vi "Scan_Hopping_CV_VUW.vi"() -> ()   [LabVIEW 2023]
uses:
  Sub_Vi/TypeDefs/Settings.ctl
  Sub_Vi/TypeDefs/ChangeOnFly.ctl
  Sub_Vi/TypeDefs/Display.ctl
  Settings.vi
panel:
  in  "Feedback Threshold \nGreater Than (Amps)":dbl=-1e-09
  in  "StopCond_GreaterThan? 2":bool
  in  "NumberOfCVsAtEachPoint":i32=1
  in  "Hopping Distance Between Lines (um)":dbl=1.0
  in  "Pre CV HoldTime /s":dbl format="%#_13g"
  in  "CV Rate / V/s":dbl=0.2
  in  "Voltage to Electrode (V) 3":dbl=-2.0
  in  "Voltage to Electrode (V) 2":dbl=1.0
  in  "Display Cluster":T1
  in  "ChangeonFly":T2
  in  "SettingsCluster":T3={"Sample Rate (us)"=1, "Samples Per Data Point (int, power of 2)"=1000, "DistanceToBulk (um)"=-1.0, "HoldTimeScaler"=40000, "SaveData"=TRUE, "DistanceToBulk (um) 2"=-1.0, "DistanceToBulk (um) 3"=-1.0}
  in  "Feedback Type":T4(ring)=enum."Current 1"
  in  "StopCond_GreaterThan?":bool=TRUE
  in  "Approach Rate Hopping (um/s)":dbl=0.15
  in  "Retract Rate (um/s)":dbl=1.0
  in  "Hopping Distance Along Line(um)":dbl=1.0
  in  "Z End (um)":dbl
  in  "Distance To Retract (um)":dbl=5.0
  in  "Upper dZ limit":i32=8
  in  "Feedback Threshold \nLess Than (Amps)":dbl=1e-09
  in  "P":fxp<+/-,32,1>=0.029999999795109034 format="%.32g"
  in  "X Center (um)":dbl=100.0 min=0.0 max=300.0
  in  "Y Center (um)":dbl=100.0 min=0.0 max=300.0
  in  "Y Width (um)":dbl=10.0
  in  "X Width (um)":dbl=10.0
  in  "Lateral Movement Rate (um/s)":dbl=5.0
  in  "Voltage to Electrode (V)":dbl=-0.4
  in  "Approach Rate (um/s)":dbl=0.5
  in  "Z Start height (um)":dbl=150.0
  in  "Start scan Button":bool
  in  "Stop":bool
  in  "Pause":bool
  out "Y end":dbl
  out "X end":dbl
  out "X start":dbl
  out "Y start":dbl
  in  "Tab Control 4":T5(tab)=enum."AC Approach 2"
  out "Topology":dbl[][](graph)
  out "Current 1":dbl[][](graph)
  out "Current 2":dbl[][](graph)
  out "Current 3":dbl[][](graph)
  out "V vs C1":cluster{"Y":dbl[], "Y":dbl[]}[](graph)
  out "Z vs C3":cluster{"Y":dbl[], "Y":dbl[]}[](graph)
  out "Lock in Phase":dbl[](graph)
  out "Lock in amp":dbl[](graph)
  out "t vs C2":dbl[](graph)
  out "t vs C1":dbl[](graph)
  out "Z vs C1":cluster{"Y":dbl[], "Y":dbl[]}[](graph)
  # "Approach  Settings"
  # "Feedback  Settings"
  # "Hopping Settings"
  # "CV"
  # "Scan  Area"
  # "Define Scan area \nAbout centre"
  # "Change top/bottom values \ndepending on scan"
  # "Change top/bottom values \ndepending on scan"
  # "Change top/bottom values \ndepending on scan"
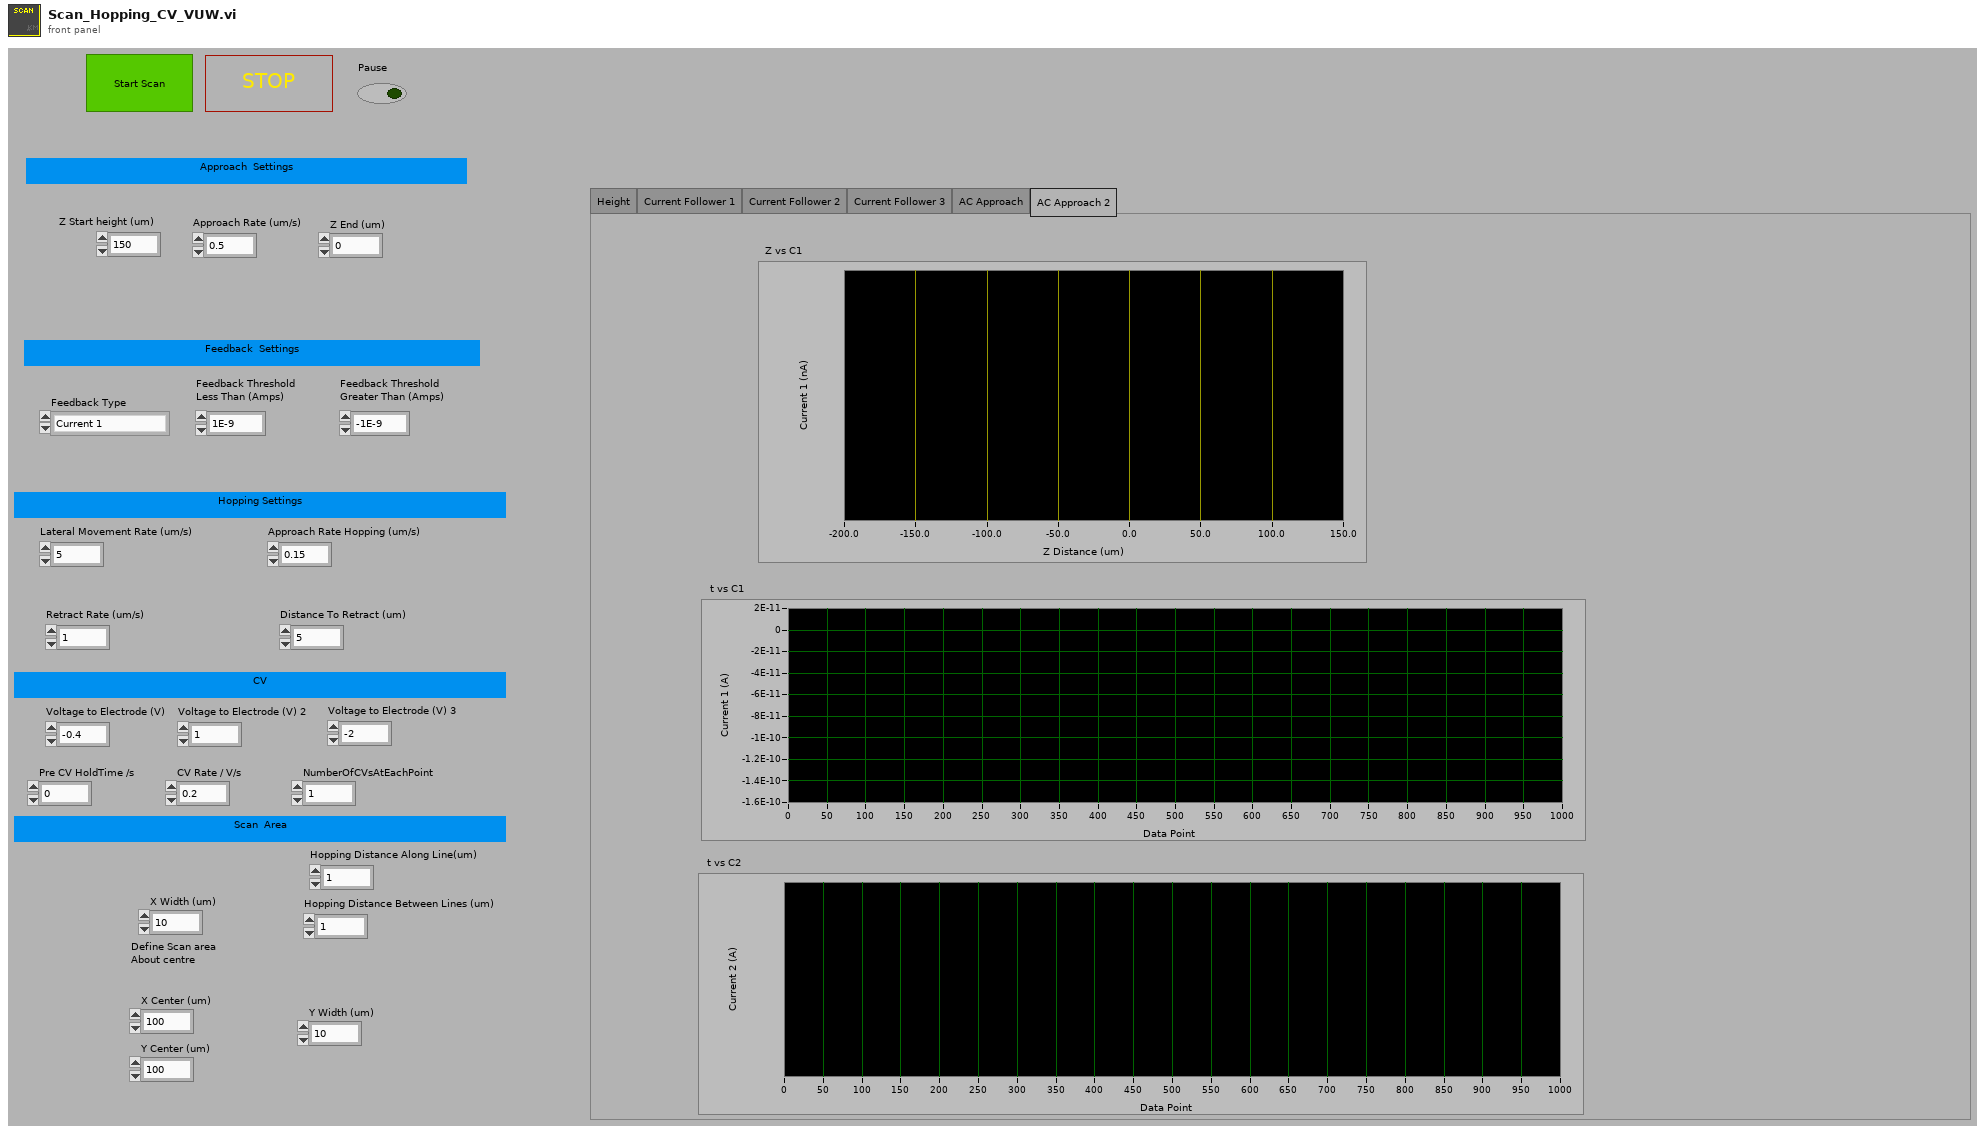
[diagram p1: front panel]
types:
  T1 = typedef "Display.ctl" = cluster{"X":refnum<vi>, "Y":refnum<vi>, "Z":refnum<vi>, "Amp":refnum<vi>, "Phase":refnum<vi>, "t vs Z":refnum<vi>, "t vs C1":refnum<vi>, "t vs C2":refnum<vi>, "t vs C3":refnum<vi>, "t vs Amp":refnum<vi>, "t vs Phase":refnum<vi>, "t vs X":refnum<vi>, "t vs Y":refnum<vi>, "Z vs C1":refnum<vi>, "Z vs C2":refnum<vi>, "Z vs C3":refnum<vi>, "V vs C1":refnum<vi>, "V vs C2":refnum<vi>, "V vs C3":refnum<vi>, "X/Y/Z F":refnum<vi>, "X/Y/Z R":refnum<vi>, "X/Y/C1 F":refnum<vi>, "X/Y/C1 R":refnum<vi>, "X/Y/C2 F":refnum<vi>, "X/Y/C2 R":refnum<vi>, "X/Y/C3 F":refnum<vi>, "X/Y/C3 R":refnum<vi>, "NumberOfLines":u16, "um Per Pixel":dbl, "um Per Line":dbl, "X Center":dbl, "Hop X/Y/Z":refnum<vi>, "Hop X/Y/C1":refnum<vi>, "Hop X/Y/C2":refnum<vi>, "Hop X/Y/C3":refnum<vi>, "X Width":dbl, "Y Width":dbl, "Hopping Distance":dbl, "V2 vs C1":refnum<vi>, "V vs Phase":refnum<vi>, "Y Center":dbl, "Number of Pixels":dbl, "V2 vs C2":refnum<vi>, "V2 vs C3":refnum<vi>, "V vs y":refnum<vi>, "V2 vs y":refnum<vi>, "Z vs Amp":refnum<vi>, "Z vs Phase":refnum<vi>}
  T2 = typedef "ChangeOnFly.ctl" = cluster{"Stop (boolean)":refnum<vi>, "Pause (boolean)":refnum<vi>, "EndCurrentLine (boolean)":refnum<vi>, "max movement per update step (Interger, nm)":refnum<vi>, "P (float, arb)":refnum<vi>, "Feedback set point (double, Amps)":refnum<vi>, "Voltage (double, V)":refnum<vi>, "Feedback set point 2 (double, Amps)":refnum<vi>, "Stop on Greater Than 2? (boolean)":refnum<vi>, "Stop on Greater Than? (boolean)":refnum<vi>, "Voltage 2 (double, V)":refnum<vi>, "Feedback Type (enum)":refnum<vi>, "Feedback Type 2 (enum)":refnum<vi>}
  T3 = typedef "Settings.ctl" = cluster{"Sample Rate (us)":u32, "Samples Per Data Point (int, power of 2)":i16, "DistanceToBulk (um)":dbl, "HoldTimeScaler":u64, "SaveData":bool, "DistanceToBulk (um) 2":dbl, "DistanceToBulk (um) 3":dbl}
  T4 = enum16{"AC Magnitude", "Current 1", "Current 2", "Phase"}
  T5 = enum32{"Height", "Current Follower 1", "Current Follower 2", "Current Follower 3", "AC Approach", "AC Approach 2"}
  T6 = cluster{"Scan Rate (um/s)":dbl, "X Start":dbl, "X End":dbl, "Y Start":dbl, "Y End":dbl, " Z Start":dbl, "HoppingDistance":dbl, "V":dbl, "Z End":dbl, "Approach Rate Hopping (um/s)":dbl, "Retrack Rate (um/s)":dbl, "V 2":dbl, "Approach Rate (um/s)":dbl, "V 3":dbl, "CV Rate / V/s":dbl, "V 4":dbl, "V 1":dbl, "HoldTime1/s":dbl, "Hold time 2 / s":dbl, "Hold time 3/ s":dbl, "HoppingDistanceBetweenLines":dbl}
  T7 = typedef "WayPointCluster.ctl" = cluster{"X (um)":dbl[], "Y (um)":dbl[], "Z (um)":dbl[], "V (V)":dbl[], "X Velocity (um s-1)":dbl[], "Y Velocity (um s-1)":dbl[], "Z Velocity (um s-1)":dbl[], "V Velocity (V s-1)":dbl[], "FeedBack Type (enum)":u16[], "Move X (boolean)":bool[], "Move Y (boolean)":bool[], "Move Z (boolean)":bool[], "Move V (boolean)":bool[], "Jump V (boolean)":bool[], "Hold (boolean)":bool[], "Hold Time":u32[], "V2 (V)":dbl[], "Move V2":bool[], "V2 Velocity (V s-1)":dbl[], "Jump V2 (boolean)":bool[], "Update z Position delta (ms)":i16[], "Hold Feedback1":bool[], "Move Z PicoMotor":bool[], " Z PicoMotor Direction":bool[], "DIO0":bool[]}
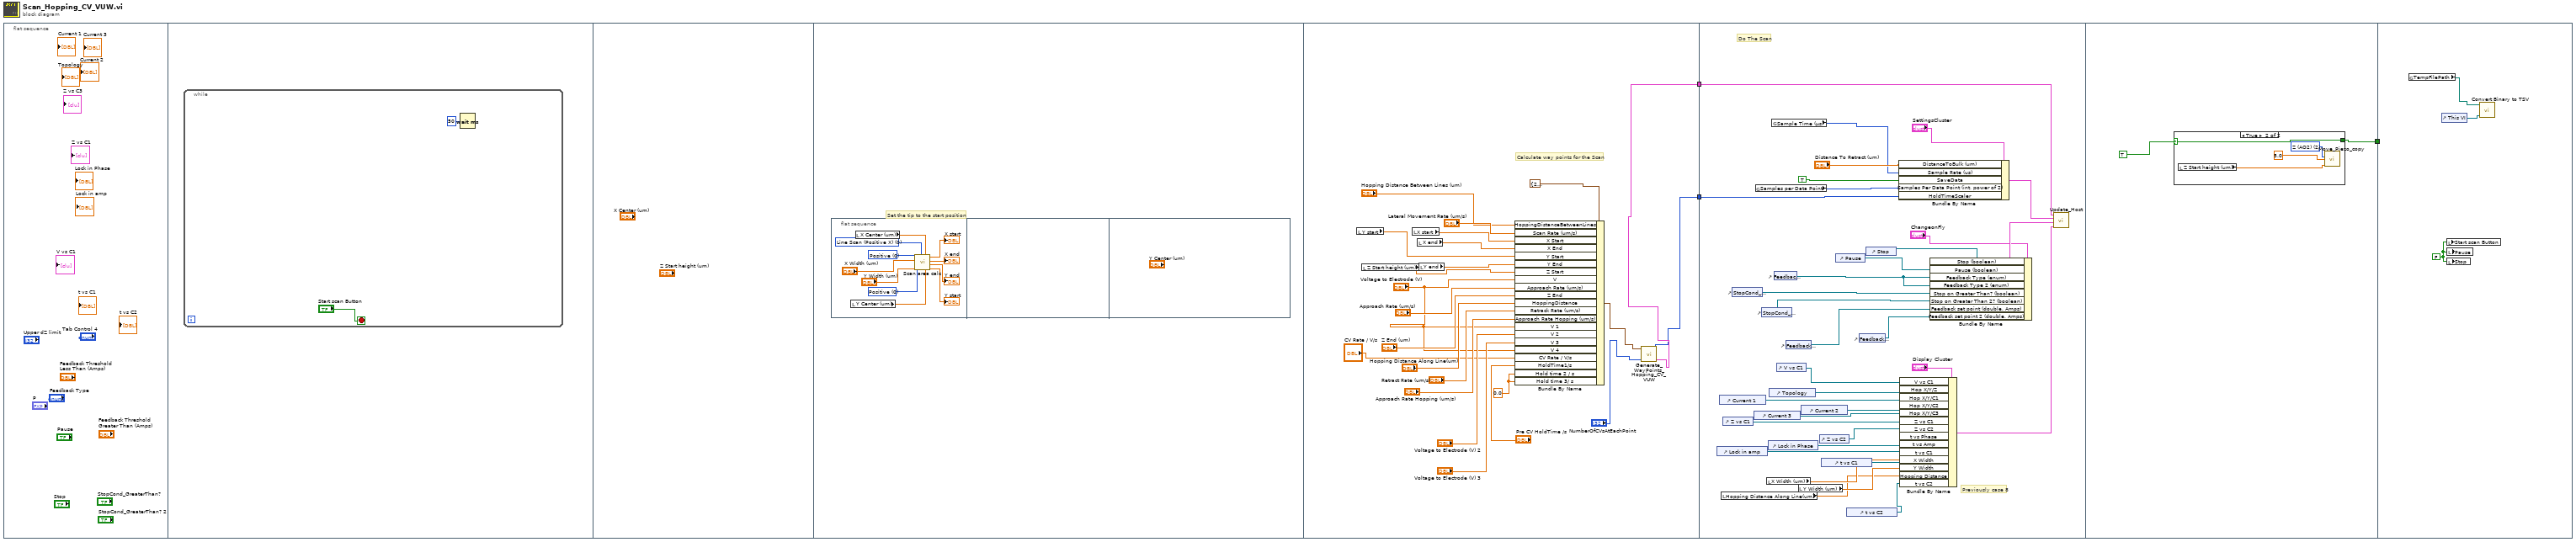
[diagram p0: block diagram]
diagram:
  n1 = flat-sequence {
    tunnel: [w18] -> w3
    tunnel: [w17] -> w1
    tunnel: w3 -> [w72]
    tunnel: w1 -> [w46]
    tunnel: [w73] -> w2
    tunnel: w2 -> [_]
    frame #0 {
    }
    frame #1 {
      n2 = while {
        stop <- "Start scan Button" stop-if-true
        n3 = Wait (ms)(milliseconds to wait=u32 50) -> ()  [unwired: 1 out]
      }
    }
    frame #2 {
    }
    frame #3 {
      # "Set the tip to the start position"
      n4 = flat-sequence {
        frame #0 {
          w6 = u16 0 items=["Positive", "Negative"] ("Major Axis Direction")
          w7 = u16 0 items=["Positive", "Negative"] ("Minor Axis Direction")
          w8 = u16 0 items=["Line Scan (Positive X)", "Line Scan (Negative X)", "Line Scan (Positive Y)", "Line Scan (Negative Y)"] ("Scan Type")
          n5 = local read "Y Center (um)"() -> (w9:dbl)
          n6 = local read "X Center (um)"() -> (w10:dbl)
          n7 = call "Scan area calc.vi"("Y Width"="Y Width (um)", "Major Axis Direction"=w6, "X Width"="X Width (um)", "Minor Axis Direction"=w7, "Scan Type"=w8, "Y Center"=w9, "X Center"=w10) -> ("Y start"=→"Y start":dbl, "Y end"=→"Y end":dbl, "X end"=→"X end":dbl, "X start"=→"X start":dbl)
        }
        frame #1 {
        }
        frame #2 {
        }
      }
    }
    frame #4 {
      w24 = 0.0 ("HoldTime1/s")
      # "Calculate way points for the Scan"
      n8 = local read "Y start"() -> (w29:dbl)
      n9 = local read "Z Start height (um)"() -> (w34:dbl)
      n10 = local read "X start"() -> (w39:dbl)
      n11 = local read "X end"() -> (w38:dbl)
      n12 = local read "Y end"() -> (w37:dbl)
      n13 = Bundle By Name(cluster=T6 {"Scan Rate (um/s)"=20.0, "X Start"=180.0, "X End"=220.0, "Y Start"=199.0, "Y End"=201.0, " Z Start"=0.0, "HoppingDistance"=0.5, "V"=0.0, "Z End"=38.0, "Approach Rate Hopping (um/s)"=0.5, "Retrack Rate (um/s)"=20.0, "V 2"=0.0, "Approach Rate (um/s)"=0.5, "V 3"=0.0, "CV Rate / V/s"=1.0, "V 4"=0.0, "V 1"=0.0, "HoldTime1/s"=0.5, "Hold time 2 / s"=0.0, "Hold time 3/ s"=0.0, "HoppingDistanceBetweenLines"=0.5} ("Input Cluster"), "HoppingDistanceBetweenLines"="Hopping Distance Between Lines (um)", "Scan Rate (um/s)"="Lateral Movement Rate (um/s)", "X Start"=w39, "X End"=w38, "Y Start"=w29, "Y End"=w37, "Z Start"=w34, "V"="Voltage to Electrode (V)", "Approach Rate (um/s)"="Approach Rate (um/s)", "Z End"="Z End (um)", "HoppingDistance"="Hopping Distance Along Line(um)", "Retrack Rate (um/s)"="Retract Rate (um/s)", "Approach Rate Hopping (um/s)"="Approach Rate Hopping (um/s)", "V 1"="Voltage to Electrode (V)", "V 2"="Voltage to Electrode (V) 2", "V 3"="Voltage to Electrode (V) 3", "V 4"="Voltage to Electrode (V)", "CV Rate / V/s"="CV Rate / V/s", "HoldTime1/s"="Pre CV HoldTime /s", "Hold time 2 / s"=w24, "Hold time 3/ s"=w24) -> (w19:T6)
      n14 = call "Generate_WayPoints_Hopping_CV_VUW.vi"("NumberOfCVsAtEachPoint"="NumberOfCVsAtEachPoint", "Input Cluster"=w19) -> ("output cluster"=w18:T7, "WaitTimeScaler"=w17:u64)  [unwired: 8 in]
    }
    frame #5 {
      # "Previously case 8"
      # "Do The Scan"
      n15 = control-ref of="Lock in amp"() -> (w65:refnum<vi>)
      n16 = control-ref of="Current 1"() -> (w59:refnum<vi>)
      n17 = local read "Hopping Distance Along Line(um)"() -> (w55:dbl)
      n18 = control-ref of="Z vs C1"() -> (w62:refnum<vi>)
      n19 = control-ref of="StopCond_GreaterThan?"() -> (w44:refnum<vi>)
      n20 = control-ref of="Current 3"() -> (w61:refnum<vi>)
      n21 = global read "Settings.vi" "Samples per Data Point"() -> (w51:u16)
      n22 = control-ref of="StopCond_GreaterThan? 2"() -> (w43:refnum<vi>)
      n23 = local read "X Width (um)"() -> (w57:dbl)
      n24 = control-ref of="Lock in Phase"() -> (w64:refnum<vi>)
      n25 = control-ref of="Topology"() -> (w58:refnum<vi>)
      n26 = global read "Settings.vi" "Sample Time (µs)"() -> (w48:u32)
      n27 = control-ref of="Feedback Type"() -> (w45:refnum<vi>)
      n28 = control-ref of="V vs C1"() -> (w49:refnum<vi>)
      n29 = control-ref of="Feedback Threshold \nLess Than (Amps)"() -> (w42:refnum<vi>)
      n30 = local read "Y Width (um)"() -> (w56:dbl)
      n31 = control-ref of="Current 2"() -> (w60:refnum<vi>)
      n32 = control-ref of="Z vs C2"() -> (w63:refnum<vi>)
      n33 = control-ref of="t vs C1"() -> (w66:refnum<vi>)
      n34 = control-ref of="Pause"() -> (w68:refnum<vi>)
      n35 = control-ref of="t vs C2"() -> (w40:refnum<vi>)
      n36 = control-ref of="Feedback Threshold \nGreater Than (Amps)"() -> (w41:refnum<vi>)
      n37 = control-ref of="Stop"() -> (w67:refnum<vi>)
      n38 = Bundle By Name(cluster="SettingsCluster", "DistanceToBulk (um)"="Distance To Retract (um)", "Sample Rate (us)"=w48, "SaveData"=TRUE ("Save Data"), "Samples Per Data Point (int, power of 2)"=w51, "HoldTimeScaler"=w46) -> (w70:T3)
      n39 = Bundle By Name(cluster="Display Cluster", "V vs C1"=w49, "Hop X/Y/Z"=w58, "Hop X/Y/C1"=w59, "Hop X/Y/C2"=w60, "Hop X/Y/C3"=w61, "Z vs C1"=w62, "Z vs C2"=w63, "t vs Phase"=w64, "t vs Amp"=w65, "t vs C1"=w66, "X Width"=w57, "Y Width"=w56, "Hopping Distance"=w55, "t vs C2"=w40) -> (w71:T1)
      n40 = Bundle By Name(cluster="ChangeonFly", "Stop (boolean)"=w67, "Pause (boolean)"=w68, "Feedback Type (enum)"=w45, "Feedback Type 2 (enum)"=w45, "Stop on Greater Than? (boolean)"=w44, "Stop on Greater Than 2? (boolean)"=w43, "Feedback set point (double, Amps)"=w42, "Feedback set point 2 (double, Amps)"=w41) -> (w69:T2)
      n41 = call "Update_Host.vi"("Display Cluster"=w71, "ChangeonFly"=w69, "SettingsCluster"=w70, "WayPointCluster"=w72) -> ()  [unwired: 6 in]
    }
    frame #6 {
      n42 = case shown="True" TRUE ("Retract after approach over (T/F)") {
        selector: TRUE ("Retract after approach over (T/F)") -> [w75 w76]
        tunnel: [w75 w76] -> w73
        frame False {
        }
        frame True {
          w79 = u16 2 items=["X (AO0)", "Y (AO1)", "Z (AO2)", "V (AO3)"] ("Channel")
          n43 = local read "Z Start height (um)"() -> (w77:dbl)
          n44 = call "Move_Piezo_copy.vi"("Piezo"=w79, "Movement Speed (µm/s)"=5.0 ("Scan Rate (um/s)"), "Position (µm) (or V)"=w77) -> ()  [unwired: 13 in]
        }
      }
    }
    frame #7 {
      w82 = FALSE ("Stop")
      n45 = global read "Settings.vi" "TempFilePath"() -> (w80:path)
      n46 = control-ref of="This VI"() -> (w81:refnum<vi>)
      n47 = local write "Start scan Button"(w82) -> ()
      n48 = local write "Pause"(w82) -> ()
      n49 = local write "Stop"(w82) -> ()
      n50 = call "Convert Binary to TSV.vi"("This VI"=w81, "TDMS DataFile Name"=w80) -> ()  [unwired: 10 in]
    }
  }
